vi "质控参数读取.vi"(7 "section":string="氨氮质控参数", 8 "error in (no error)":errorcluster caption="错误输入（无错误）") -> (0 "error out":errorcluster caption="错误输出", 3 "参数":T1)   [LabVIEW 2016, in "质控单元.lvlib"]
uses:
  <vilib>/Utility/config.llb/Read Key (Double).vi
  <vilib>/Utility/config.llb/NI_LVConfig.lvlib
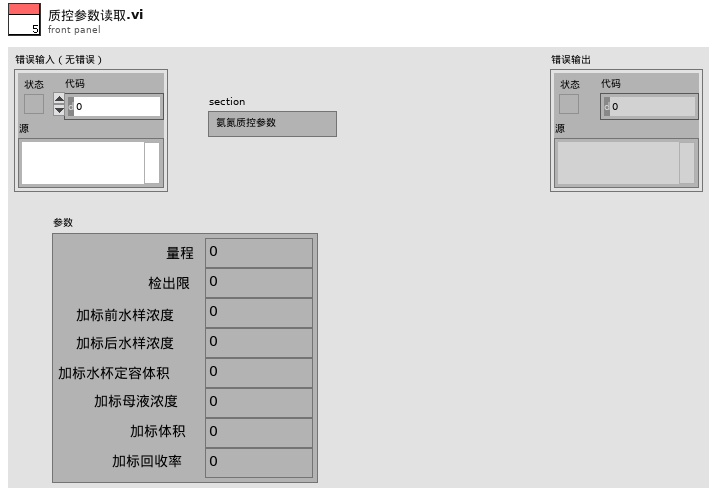
[diagram p1: front panel]
types:
  T1 = cluster{"量程":dbl, "检出限":dbl, "加标前水样浓度":dbl, "加标后水样浓度":dbl, "加标水杯定容体积":dbl, "加标母液浓度":dbl, "加标体积":dbl, "加标回收率":dbl}
  T2 = typedef "NI_LVConfig.lvlib/Config Data RefNum.ctl" = refnum<k1>
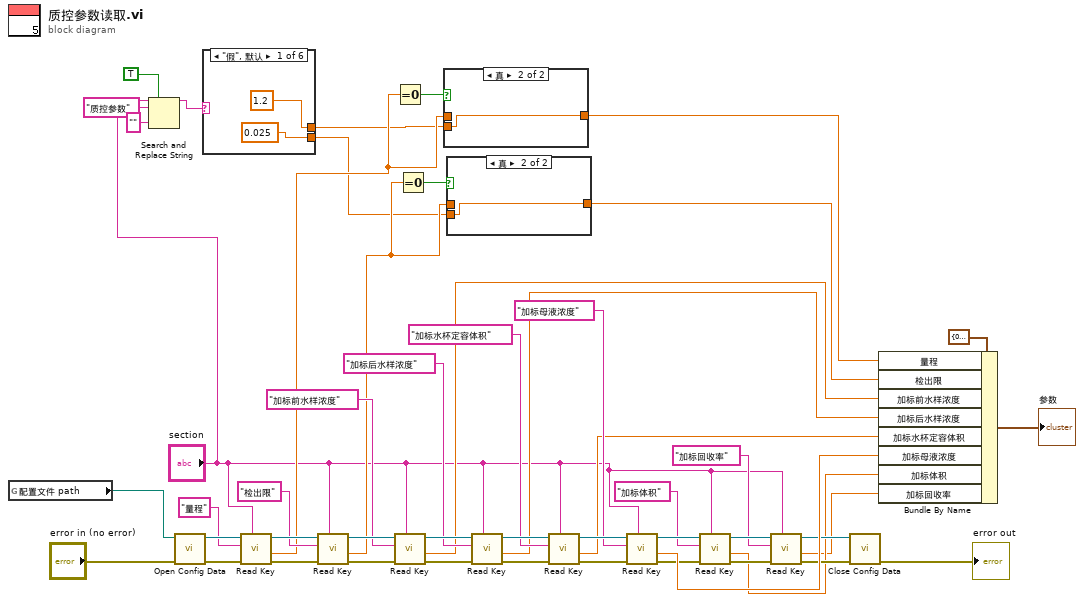
[diagram p0: block diagram]
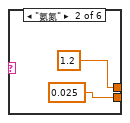
[diagram p2: hidden frame]
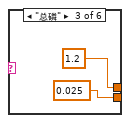
[diagram p3: hidden frame]
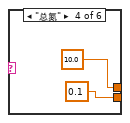
[diagram p4: hidden frame]
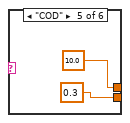
[diagram p5: hidden frame]
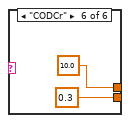
[diagram p6: hidden frame]
diagram:
  n1 = global read "质控内部交互全局.vi" "配置文件 path"() -> (w8:path)
  n2 = Search and Replace String(replace all?=TRUE ("替换全部？(F)"), input string="section", search string="质控参数" ("搜索字符串"), replace string="" ("替换字符串(\"\")")) -> (result string=w3:string)  [unwired: 4 in, 3 out]
  n3 = call <vilib>:"Open Config Data.vi"("error in (no error)"="error in (no error)", "configuration file path"=w8) -> ("error out"=w49:errorcluster, "refnum"=w50:T2)  [unwired: 7 in, 1 out]
  n4 = case shown="\"假\", 默认" w3 {
    tunnel: [1.2 ("value") 1.2 ("value") 1.2 ("value") 10.0 ("value") 10.0 ("value") 10.0 ("value")] -> w2
    tunnel: [0.025 ("value") 0.025 ("value") 0.025 ("value") 0.1 ("value") 0.3 ("value") 0.3 ("value")] -> w1
    frame "假", Default {
    }
    frame "氨氮" {
    }
    frame "总磷" {
    }
    frame "总氮" {
    }
    frame "COD" {
    }
    frame "CODCr" {
    }
  }
  n5 = call-poly <vilib>:"Read Key.vi"("section"="section", "error in (no error)"=w49, "key"="量程", "refnum"=w50) -> ("error out"=w46:errorcluster, "value"=w13:dbl, "refnum out"=w47:T2)  [unwired: 4 in, 1 out]
  n6 = call-poly <vilib>:"Read Key.vi"("section"="section", "error in (no error)"=w46, "key"="检出限", "refnum"=w47) -> ("error out"=w44:errorcluster, "value"=w10:dbl, "refnum out"=w45:T2)  [unwired: 4 in, 1 out]
  n7 = Equal To 0?(x=w13) -> (x = 0?=w14:bool)
  n8 = call-poly <vilib>:"Read Key.vi"("section"="section", "error in (no error)"=w44, "key"="加标前水样浓度", "refnum"=w45) -> ("error out"=w38:errorcluster, "value"=w32:dbl, "refnum out"=w39:T2)  [unwired: 4 in, 1 out]
  n9 = Equal To 0?(x=w10) -> (x = 0?=w11:bool)
  n10 = case shown="真" w14 {
    tunnel: w13 -> [w63 _]
    tunnel: [w63 w64] -> w12
    tunnel: w2 -> [_ w64]
    frame False {
    }
    frame True {
    }
  }
  n11 = case shown="真" w11 {
    tunnel: w10 -> [w65 _]
    tunnel: [w65 w66] -> w9
    tunnel: w1 -> [_ w66]
    frame False {
    }
    frame True {
    }
  }
  n12 = call-poly <vilib>:"Read Key.vi"("section"="section", "error in (no error)"=w38, "key"="加标后水样浓度", "refnum"=w39) -> ("error out"=w41:errorcluster, "value"=w31:dbl, "refnum out"=w40:T2)  [unwired: 4 in, 1 out]
  n13 = call-poly <vilib>:"Read Key.vi"("section"="section", "error in (no error)"=w41, "key"="加标水杯定容体积", "refnum"=w40) -> ("error out"=w43:errorcluster, "value"=w30:dbl, "refnum out"=w42:T2)  [unwired: 4 in, 1 out]
  n14 = call-poly <vilib>:"Read Key.vi"("section"="section", "error in (no error)"=w43, "key"="加标母液浓度", "refnum"=w42) -> ("error out"=w21:errorcluster, "value"=w29:dbl, "refnum out"=w23:T2)  [unwired: 4 in, 1 out]
  n15 = call-poly <vilib>:"Read Key.vi"("section"="section", "error in (no error)"=w21, "key"="加标体积", "refnum"=w23) -> ("error out"=w20:errorcluster, "value"=w18:dbl, "refnum out"=w24:T2)  [unwired: 4 in, 1 out]
  n16 = call-poly <vilib>:"Read Key.vi"("section"="section", "error in (no error)"=w20, "key"="加标回收率", "refnum"=w24) -> ("error out"=w19:errorcluster, "value"=w17:dbl, "refnum out"=w22:T2)  [unwired: 4 in, 1 out]
  n17 = call <vilib>:"Close Config Data.vi"("error in (no error)"=w19, "refnum"=w22) -> ("error out"=→"error out":errorcluster)  [unwired: 8 in, 1 out]
  n18 = Bundle By Name(cluster=T1 {"量程"=0.0, "检出限"=0.0, "加标前水样浓度"=0.0, "加标后水样浓度"=0.0, "加标水杯定容体积"=0.0, "加标母液浓度"=0.0, "加标体积"=0.0, "加标回收率"=0.0} ("参数"), "量程"=w12, "检出限"=w9, "加标前水样浓度"=w32, "加标后水样浓度"=w31, "加标水杯定容体积"=w30, "加标母液浓度"=w29, "加标体积"=w18, "加标回收率"=w17) -> (→"参数":T1)
